vi "Wait for Data Availability.vi"(8 "error in":errorcluster, 9 "Time out":i32, 10 "Samples to read":u32) -> (0 "error out":errorcluster, 2 "Data out":u32[][](array[numeric]))   [LabVIEW 2021]
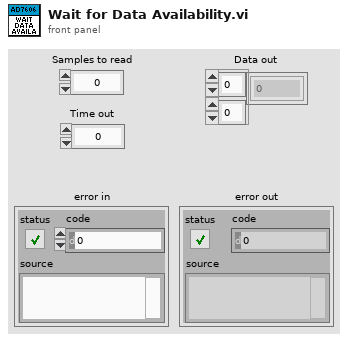
[diagram p1: front panel]
types:
  T1 = enum16{"Initialize", "Write", "Read", "GetBacklog", "Reset"}
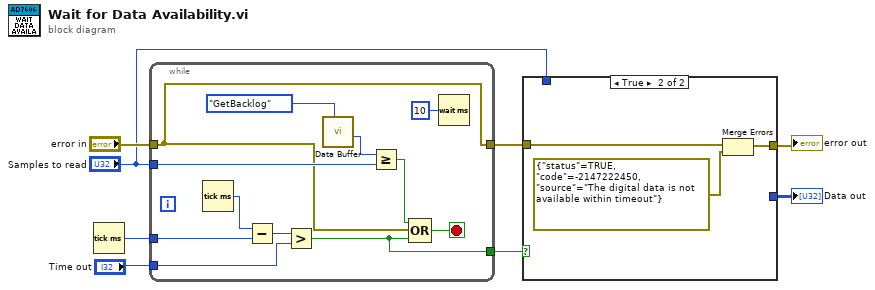
[diagram p0: block diagram]
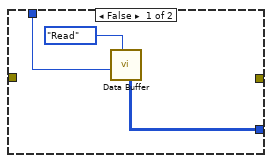
[diagram p2: hidden frame]
diagram:
  n1 = Tick Count (ms)() -> (millisecond timer value=w8:u32)
  n2 = while {
    tunnel: w8 -> [w18]
    tunnel: "Time out" -> [w16]
    tunnel: "Samples to read" -> [w15]
    tunnel: [w12] -> w6
    tunnel: "error in" -> [w9]
    tunnel: [w9] -> w1
    stop <- w13 stop-if-true
    n3 = Tick Count (ms)() -> (millisecond timer value=w19:u32)
    n4 = Subtract(x=w19, y=w18) -> (x-y=w17:u32)
    n5 = Greater?(x=w17, y=w16) -> (0:w12:bool)
    n6 = call "Data Buffer.vi"("Operation"=T1."GetBacklog") -> ("Elements remaining"=w11:u32)  [unwired: 9 in, 1 out]
    n7 = Greater Or Equal?(x=w11, y=w15) -> (x >= y?=w10:bool)
    n8 = Compound Arithmetic op=OR(w10, w9, w12) -> (w13:bool)
    n9 = Wait (ms)(milliseconds to wait=u32 10) -> ()  [unwired: 1 out]
  }
  n10 = case shown="True" w6 {
    tunnel: "Samples to read" -> [w22 _]
    tunnel: [w21 _] -> w4
    tunnel: [_ w26] -> w3
    tunnel: w1 -> [_ w24]
    frame False {
      n11 = call "Data Buffer.vi"("Operation"=T1."Read", "Samples to read"=w22) -> ("Data out"=w21:u32[][])  [unwired: 8 in, 1 out]
    }
    frame True {
      n12 = Merge Errors(w24, errorcluster {"status"=TRUE, "code"=-2147222450, "source"="The digital data is not available within timeout"} ("error in")) -> (w26:errorcluster)
    }
  }
  "Data out" <- w4
  "error out" <- w3
